vi "Measure And Log Main.vi"() -> ()   [LabVIEW 2023]
doc: "This template is for the Queued Message Handler design pattern.\n\nThe Event Handling Loop generates messages based on user interface actions.\n\nThe Message Handling Loop processes messages generated by the Event Handling Loop, or by other messages. The messages are string values, so new messages can be added easily to the Message Cases case structure in the Message Handling Loop. Each message cluster can also provide an optional value for Message Data, which is a variant that can be converted to whatever message-specific data is required."
uses:
  messages/MeasureAndLogMessage.lvclass/MeasureAndLogMessage.ctl
  <extravilib>/ChannelInstances/Lossy Stream-a[.](wfm(dbl))/Read With Abort.vi
  <extravilib>/ChannelInstances/Stream-str/Read With Abort.vi
  <extravilib>/ChannelInstances/Messenger-class'MeasureAndLogMessage'/Write With Abort.vi
  <extravilib>/ChannelInstances/Lossy Stream-a[.](wfm(dbl))/EndpointRead.vi
  <extravilib>/ChannelInstances/Stream-str/EndpointRead.vi
  <extravilib>/ChannelInstances/Tag-bool/Instantiate.vi
  <extravilib>/ChannelInstances/Stream-str/Instantiate.vi
  <extravilib>/ChannelInstances/Stream-str/)Channel.vi
  <resource>/ChannelSupport/_ChannelSupport/WaitIfNeeded.vi
  <extravilib>/ChannelInstances/Tag-t'Measure and Log Settings.ctl'/Instantiate.vi
  <extravilib>/ChannelInstances/Stream-a[.](wfm(dbl))/Instantiate.vi
  <extravilib>/ChannelInstances/Lossy Stream-a[.](wfm(dbl))/Instantiate.vi
  <extravilib>/ChannelInstances/Lossy Stream-a[.](wfm(dbl))/)Channel.vi
  <extravilib>/ChannelInstances/Tag-path/Instantiate.vi
  <extravilib>/ChannelInstances/Messenger-class'MeasureAndLogMessage'/Instantiate.vi
  <extravilib>/ChannelInstances/Messenger-class'MeasureAndLogMessage'/Endpoint.vi
  messages/MeasureAndLogMessage.lvclass
  <extravilib>/ChannelInstances/Stream-str.lvlib
  <extravilib>/ChannelInstances/Lossy Stream-a[.](wfm(dbl)).lvlib
  <extravilib>/ChannelInstances/Messenger-class'MeasureAndLogMessage'.lvlib
panel:
  in  "Exit flag":bool
  in  "Record":bool
  in  "Stop":bool
  out "Data":waveform(dbl)[](graph)
  out "Status":string
  in  "Settings":bool
  in  "Start":bool
  in  "Exit":bool
  # "Continuous Measurement Data Logger"
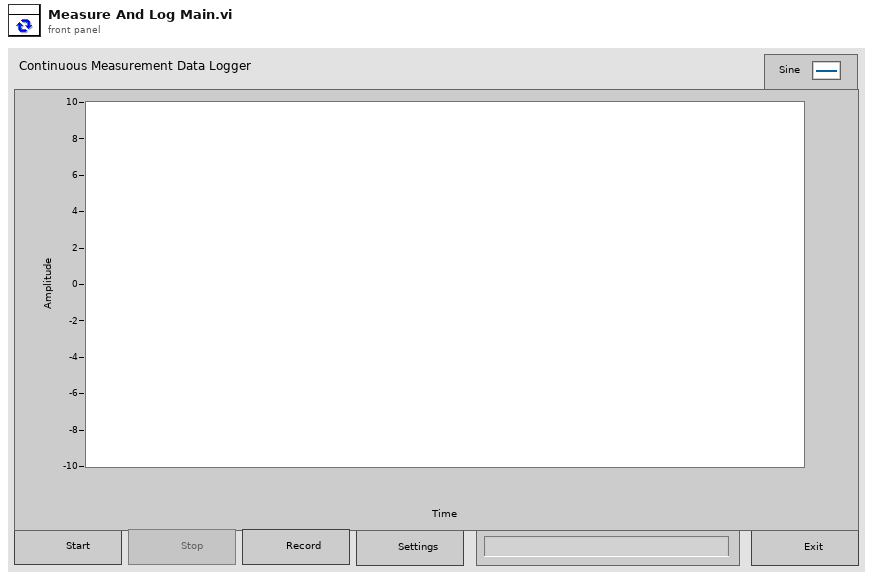
[diagram p1: front panel]
types:
  T1 = typedef "Measure and Log Settings.ctl" = cluster{"sample rate":dbl, "input range":dbl, "logfile path":path, "Simulated Signal":cluster{"signal type":T2, "frequency":dbl, "amplitude":dbl}}
  T2 = typedef "Simulated Signal Type.ctl" = enum16{"Sine Wave", "Square Wave with Noise"}
  T3 = enum8{"Enabled", "Disabled", "Disabled and Grayed Out"}
  T4 = typedef "Messenger-class'MeasureAndLogMessage'.lvlib/))Channel.ctl" = refnum<queue>
  T5 = typedef "Stream-str.lvlib/)Channel.ctl" = refnum<queue>
  T6 = typedef "Lossy Stream-a[.](wfm(dbl)).lvlib/)Channel.ctl" = refnum<queue>
  T7 = typedef "Tag-bool.lvlib/))Channel.ctl" = refnum<queue>
  T8 = typedef "Stream-a[.](wfm(dbl)).lvlib/)Channel.ctl" = refnum<queue>
  T9 = typedef "Tag-t'Measure and Log Settings.ctl'.lvlib/))Channel.ctl" = refnum<queue>
  T10 = typedef "Tag-path.lvlib/))Channel.ctl" = refnum<queue>
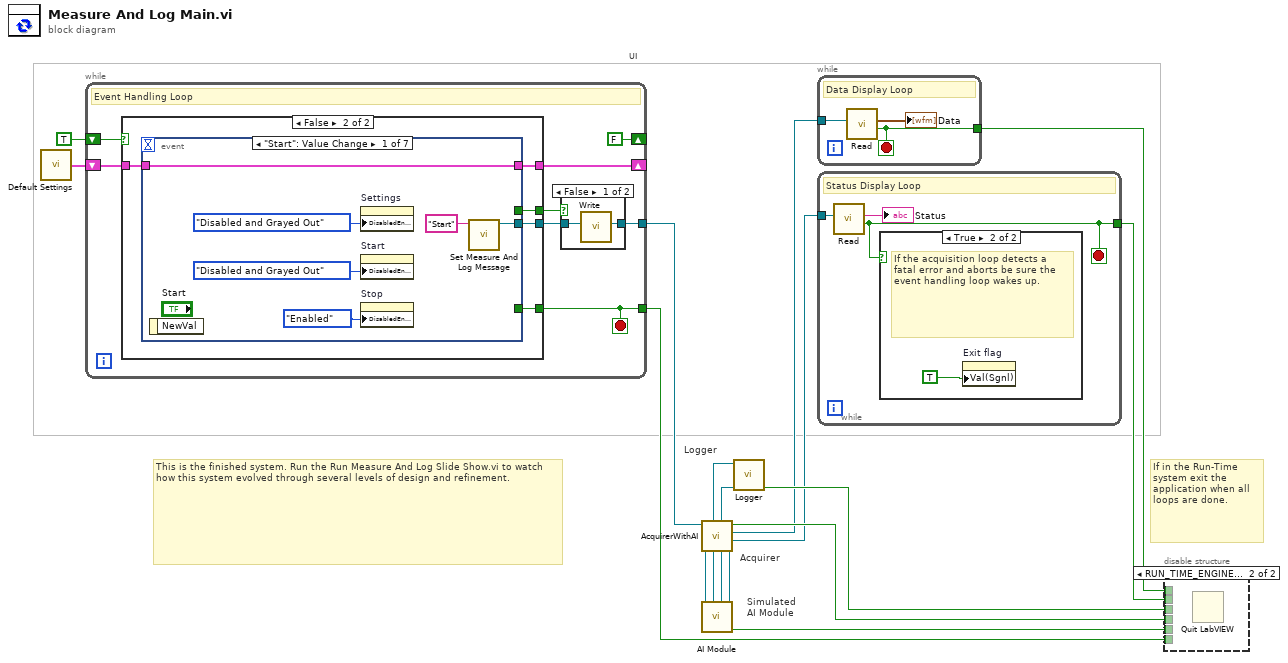
[diagram p0: block diagram]
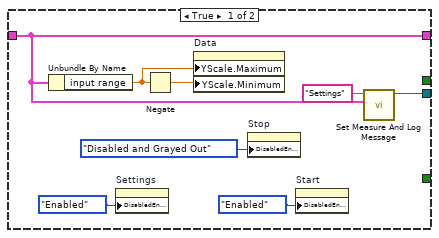
[diagram p2: hidden frame]
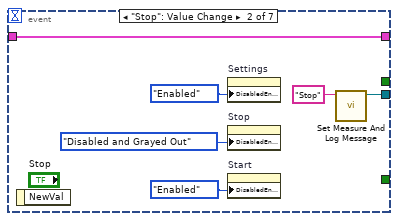
[diagram p3: hidden frame]
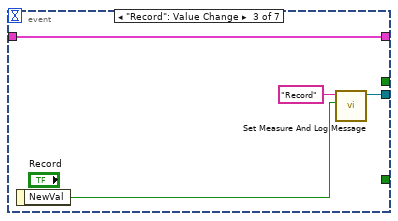
[diagram p4: hidden frame]
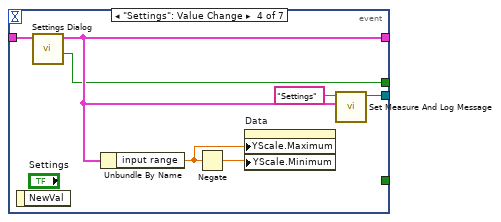
[diagram p5: hidden frame]
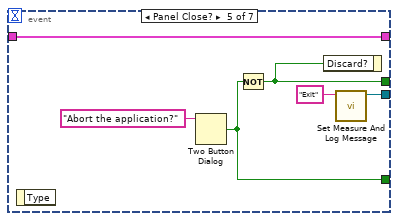
[diagram p6: hidden frame]
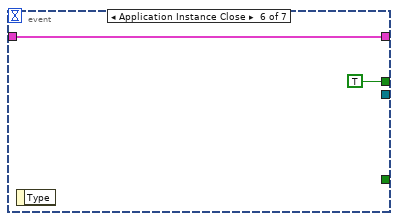
[diagram p7: hidden frame]
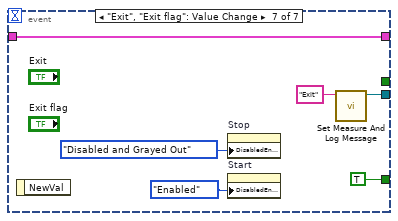
[diagram p8: hidden frame]
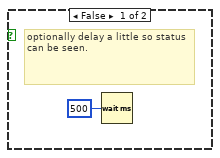
[diagram p10: hidden frame]
diagram:
  # "This is the finished system. Run the Run Measure And Log Slide Show.vi to watch how this system evolved through several levels of design and refinement."
  # "If in the Run-Time system exit the application when all loops are done."
  # "Simulated\nAI Module"
  # "Logger"
  # "Acquirer"
  # "UI"
  n1 = call "Default Settings.vi"() -> ("default settings"=w14:T1)
  n2 = while {
    tunnel: [w22] -> w12
    tunnel: [w25] -> w17
    shift-right: [w24] -> _
    shift-left: w14 -> [w23]
    shift-right: [FALSE] -> _
    shift-left: TRUE -> [w19]
    stop <- w25 stop-if-true
    # "Event Handling Loop"
    n3 = case shown="False" w19 {
      tunnel: [_ w38] -> w25
      tunnel: [w32 w37] -> w24
      tunnel: w23 -> [w32 w36]
      tunnel: [w28 w35] -> w21
      tunnel: [_ w34] -> w20
      frame True {
        n4 = Unbundle By Name(w32) -> ("input range"=w26:dbl)
        n5 = property on="Settings" class="Bool"("DisabledEnum"=T3."Enabled" ("Disabled")) -> ()  [unwired: 2 in, 2 out]
        n6 = Negate(x=w26) -> (-x=w27:dbl)
        n7 = property on="Data" class="WFChart (strict)"("YScale.Maximum"=w26, "YScale.Minimum"=w27) -> ()  [unwired: 2 in, 2 out]
        n8 = property on="Stop" class="Bool"("DisabledEnum"=T3."Disabled and Grayed Out" ("Disabled")) -> ()  [unwired: 2 in, 2 out]
        n9 = property on="Start" class="Bool"("DisabledEnum"=T3."Enabled" ("Disabled")) -> ()  [unwired: 2 in, 2 out]
        n10 = call "Set Measure And Log Message.vi"("args"=w32, "command"="Settings") -> ("MyMessage"=w28:refnum<class "MeasureAndLogMessage.lvclass">)  [unwired: 9 in]
      }
      frame False {
        n11 = event shown="[0] \"Start\": Value Change" {
          selector: _ -> [_ _ _ _ _ _ _]
          dyn-events: _ -> [_ _ _ _ _ _ _]
          timeout: _ -> [_ _ _ _ _ _ _]
          tunnel: [_ _ _ _ w63 _ TRUE] -> w38
          tunnel: [w40 w46 w52 w60 w66 w69 w71] -> w37
          tunnel: w36 -> [w40 w46 w52 w61 w66 w69 w71]
          tunnel: [w39 w45 w51 w59 w64 _ w70] -> w35
          tunnel: [_ _ _ w57 w62 TRUE ("cancelled") _] -> w34
          event "Start": Value Change {
            n12 = event-data() -> ()  [unwired: 1 in, 1 out]
            n13 = property on="Settings" class="Bool"("DisabledEnum"=T3."Disabled and Grayed Out" ("Disabled")) -> ()  [unwired: 2 in, 2 out]
            n14 = property on="Start" class="Bool"("DisabledEnum"=T3."Disabled and Grayed Out" ("Disabled")) -> ()  [unwired: 2 in, 2 out]
            n15 = property on="Stop" class="Bool"("DisabledEnum"=T3."Enabled" ("Disabled")) -> ()  [unwired: 2 in, 2 out]
            n16 = call "Set Measure And Log Message.vi"("command"="Start") -> ("MyMessage"=w39:refnum<class "MeasureAndLogMessage.lvclass">)  [unwired: 10 in]
          }
          event "Stop": Value Change {
            n17 = event-data() -> ()  [unwired: 1 in, 1 out]
            n18 = property on="Settings" class="Bool"("DisabledEnum"=T3."Enabled" ("Disabled")) -> ()  [unwired: 2 in, 2 out]
            n19 = property on="Stop" class="Bool"("DisabledEnum"=T3."Disabled and Grayed Out" ("Disabled")) -> ()  [unwired: 2 in, 2 out]
            n20 = property on="Start" class="Bool"("DisabledEnum"=T3."Enabled" ("Disabled")) -> ()  [unwired: 2 in, 2 out]
            n21 = call "Set Measure And Log Message.vi"("command"="Stop") -> ("MyMessage"=w45:refnum<class "MeasureAndLogMessage.lvclass">)  [unwired: 10 in]
          }
          event "Record": Value Change {
            n22 = event-data() -> ("NewVal"=w53:bool)  [unwired: 1 in]
            n23 = call "Set Measure And Log Message.vi"("args"=w53, "command"="Record") -> ("MyMessage"=w51:refnum<class "MeasureAndLogMessage.lvclass">)  [unwired: 9 in]
          }
          event "Settings": Value Change {
            n24 = event-data() -> ()  [unwired: 1 in, 1 out]
            n25 = call "Settings Dialog.vi"("settings in"=w61) -> ("cancelled"=w57:bool, "settings out"=w60:T1)  [unwired: 9 in]
            n26 = Unbundle By Name(w60) -> ("input range"=w55:dbl)
            n27 = Negate(x=w55) -> (-x=w56:dbl)
            n28 = property on="Data" class="WFChart (strict)"("YScale.Maximum"=w55, "YScale.Minimum"=w56) -> ()  [unwired: 2 in, 2 out]
            n29 = call "Set Measure And Log Message.vi"("args"=w60, "command"="Settings") -> ("MyMessage"=w59:refnum<class "MeasureAndLogMessage.lvclass">)  [unwired: 9 in]
          }
          event Panel Close? {
            n30 = event-data() -> ()  [unwired: 1 in, 1 out]
            n31 = Two Button Dialog(message="Abort the application?") -> (T button?=w63:bool)  [unwired: 2 in]
            n32 = Not(x=w63) -> (.not. x?=w62:bool)
            n33 = event-data("Discard?"=w62) -> ()  [unwired: 1 in, 1 out]
            n34 = call "Set Measure And Log Message.vi"("command"="Exit") -> ("MyMessage"=w64:refnum<class "MeasureAndLogMessage.lvclass">)  [unwired: 10 in]
          }
          event Application Instance Close {
            n35 = event-data() -> ()  [unwired: 1 in, 1 out]
          }
          event "Exit", "Exit flag": Value Change {
            n36 = event-data() -> ()  [unwired: 1 in, 1 out]
            n37 = property on="Stop" class="Bool"("DisabledEnum"=T3."Disabled and Grayed Out" ("Disabled")) -> ()  [unwired: 2 in, 2 out]
            n38 = property on="Start" class="Bool"("DisabledEnum"=T3."Enabled" ("Disabled")) -> ()  [unwired: 2 in, 2 out]
            n39 = call "Set Measure And Log Message.vi"("command"="Exit") -> ("MyMessage"=w70:refnum<class "MeasureAndLogMessage.lvclass">)  [unwired: 10 in]
          }
        }
      }
    }
    n40 = case shown="False" w20 {
      tunnel: [w77 _] -> w22
      tunnel: w21 -> [w76 _]
      frame False {
        n41 = call <extravilib>:"Write.vi"("element"=w76) -> ("channel"=w77:T4)  [unwired: 8 in, 2 out]
      }
      frame True {
      }
    }
  }
  n42 = call "AcquirerWithAI.vi"("waveform data"=w4, "command stream"=w12) -> ("status stream"=w2:T5, "wfm data lossy stream"=w5:T6, "done"=w7:bool, "start/stop"=w1:T7, "wfm data stream"=w6:T8, "settings"=w3:T9, "file path tag"=w8:T10, "exit"=w9:T7)  [unwired: 2 in]
  n43 = call "AI Module.vi"("acquire tag"=w1, "configuration tag"=w3, "exit tag"=w9) -> ("done"=w10:bool, "wfm data stream"=w4:T8)  [unwired: 7 in]
  n44 = call "Logger.vi"("wfm data stream"=w6, "file path tag"=w8) -> ("done"=w11:bool)  [unwired: 9 in]
  n45 = while {
    tunnel: [w80] -> w15
    tunnel: w5 -> [w78]
    stop <- w80 stop-if-true
    # "Data Display Loop"
    n46 = call <extravilib>:"Read.vi"("channel"=w78) -> ("last element?"=w80:bool, "element"=→"Data":waveform(dbl)[])  [unwired: 5 in, 4 out]
  }
  n47 = while {
    tunnel: w2 -> [w83]
    tunnel: [w81] -> w16
    stop <- w81 stop-if-true
    # "Status Display Loop"
    n48 = call <extravilib>:"Read.vi"("channel"=w83) -> ("last element?"=w81:bool, "element"=→"Status":string)  [unwired: 6 in, 3 out]
    n49 = case shown="True" w81 {
      frame False {
        # "optionally delay a little so status can be seen."
        n50 = Wait (ms)(milliseconds to wait=u32 500) -> ()  [unwired: 1 out]
      }
      frame True {
        # "If the acquisition loop detects a fatal error and aborts be sure the event handling loop wakes up."
        n51 = property on="Exit flag" class="Bool (strict)"("Val(Sgnl)"=TRUE) -> ()  [unwired: 2 in, 2 out]
      }
    }
  }
  n52 = disable-structure shown="RUN_TIME_ENGINE==True" {
    disable-tunnel: w17 -> [_ _]
    disable-tunnel: w16 -> [_ _]
    disable-tunnel: w15 -> [_ _]
    disable-tunnel: w10 -> [_ _]
    disable-tunnel: w11 -> [_ _]
    disable-tunnel: w7 -> [_ _]
    frame condition #0 (active) {
    }
    frame condition #1 {
      n53 = Quit LabVIEW() -> ()  [unwired: 1 in]
    }
  }
